vi "Read RawData.vi"(8 "error in (no error)":errorcluster, 9 "WCM_max_value":bool, 10 "# of scans":i32, 11 "Detector in":refnum<class "Detector.lvclass">) -> (0 "error out":errorcluster, 1 "Channel II":i32[][](array[numeric]), 2 "Channel I":i32[][](array[numeric]), 3 "Detector out":refnum<class "Detector.lvclass">, 4 "WCM_values":sgl[](array[numeric]))   [LabVIEW 2015, in "Detector.lvclass"]
uses:
  Detector.lvclass
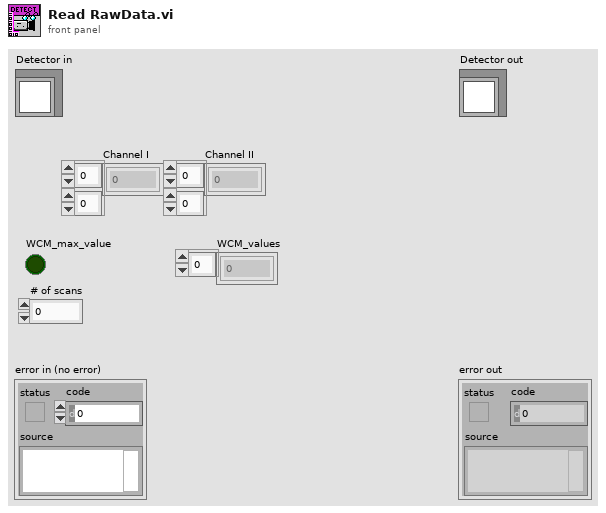
[diagram p1: front panel]
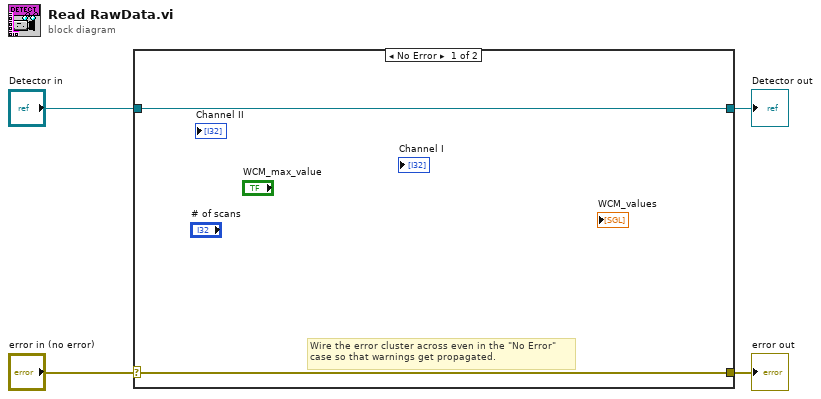
[diagram p0: block diagram]
diagram:
  n1 = case shown="No Error" "error in (no error)" {
    selector: "error in (no error)" -> [w5 w8]
    tunnel: [w5 w8] -> w3
    tunnel: [w6 w7] -> w1
    tunnel: "Detector in" -> [w6 w7]
    frame No Error {
      # "Wire the error cluster across even in the \"No Error\"\ncase so that warnings get propagated."
    }
    frame Error {
    }
  }
  "error out" <- w3
  "Detector out" <- w1
